vi "Waveform - Append.vi"() -> ()   [LabVIEW 2023]
doc: "Shows how to append two waveforms."
uses:
  <vilib>/Waveform/WDTOps.llb/WDT Append Waveforms DBL.vi
panel:
  out "Appended Waveforms":waveform(dbl)(graph)
  out "Initial Waveforms":waveform(dbl)[](graph)
  # "Overview: Demonstrates how to append one waveform to another waveform with the Append Waveforms VI.\nInstructions:\nRun the VI. The sawtooth waveform will be appended to the end of the sine waveform."
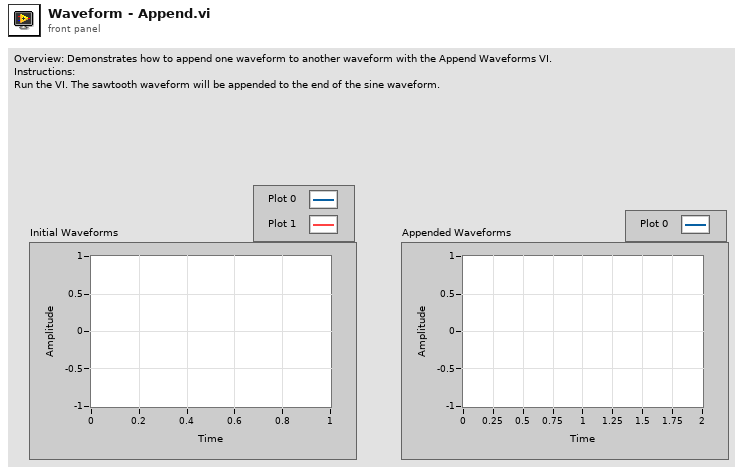
[diagram p1: front panel]
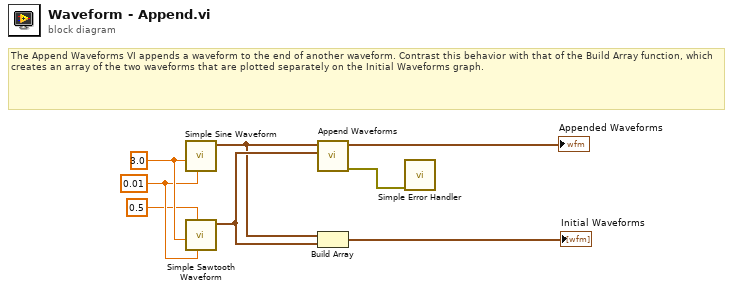
[diagram p0: block diagram]
diagram:
  w5 = 0.01
  w6 = 3.0
  # "The Append Waveforms VI appends a waveform to the end of another waveform. Contrast this behavior with that of the Build Array function, which creates an array of the two waveforms that are plotted separately on the Initial Waveforms graph."
  n1 = call "Simple Sine Waveform.vi"("delta t"=w5, "n cycles"=w6) -> ("sine waveform"=w7:waveform(dbl))  [unwired: 9 in]
  n2 = call "Simple Sawtooth Waveform.vi"("delta t"=w5, "amplitude"=0.5, "n cycles"=w6) -> ("sawtooth waveform"=w8:waveform(dbl))  [unwired: 8 in]
  n3 = call-poly <vilib>:"Append Waveforms.vi"("waveform B"=w8, "waveform A"=w7) -> ("error out"=w3:errorcluster, "waveform out"=→"Appended Waveforms":waveform(dbl))  [unwired: 8 in]
  n4 = Build Array "Build Array"(w7, w8) -> (→"Initial Waveforms":waveform(dbl)[])
  n5 = call <vilib>:"Simple Error Handler.vi"("error in (no error)"=w3) -> ()  [unwired: 4 in, 5 out]
